vi "ShooterSpeedRegulateV2.vi"(0 "Shooter Speed":T1(ring)) -> (4 "ALL GOOD":bool, 10 "Motor 1 Output":dbl)   [LabVIEW 2012]
uses:
  Robot Global Data.vi
  Max'sToolKit/ConvertVoltageToPercentVbs.vi
  <vilib>/addons/control/pid/pid.llb/PID (DBL).vi
  <vilib>/addons/control/pid/NI_PID_pid.lvlib
panel:
  in  "Reset Shooter PID":bool
  out "Loop Rate (Hz)":dbl
  out "Array Index":dbl
  out "Wheel 1 RPS":dbl
  out "W1 Target RPS":dbl
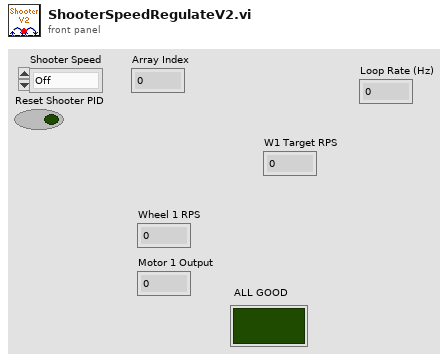
[diagram p1: front panel]
types:
  T1 = enum16{"Off", "2pt Key Shot", "3pt Key Shot", "Back Shot", "Fender Shot", "Key Close", "Key Far"}
  T2 = typedef "WPI_EncoderDevRef.ctl" = cluster{"DevStatus":errorcluster, "EncoderIndex":T3, "CounterIndex":T4, "DistancePerCount":dbl, "Decoding Type":T5}
  T3 = typedef "FPGA_EncoderIdx.ctl" = enum8{"Enc 0", "Enc 1", "Enc 2", "Enc 3", "Invalid"}
  T4 = typedef "FPGA_CounterCtrSystemIndex.ctl" = enum8{"Ctr 0", "Ctr 1", "Ctr 2", "Ctr 3", "Ctr 4", "Ctr 5", "Ctr 6", "Ctr 7", "Invalid"}
  T5 = typedef "WPI_EncoderType.ctl" = enum16{"1x", "2x", "4x"}
  T6 = cluster{"proportional gain (Kc)":dbl, "integral time (Ti, min)":dbl, "derivative time (Td, min)":dbl}
  T7 = typedef "WPI_MotorControlDeviceRef.ctl" = cluster{"DeviceStatus":errorcluster, "Type":enum16{"PWM", "CAN"}, "PWM":cluster{"Digital Module":T8, "PWM Channel":T9, "DeadBand":T10}, "CAN":cluster{"Device Number":u8, "Control Mode":T11, "Semaphore":T12, "Max Vout":dbl}, "Invert":bool, "TransformRef":T13, "InvTransformRef":T13}
  T8 = typedef "FPGA_TypedefDigitalModule.ctl" = enum16{"Digital Module 1", "Digital Module 2"}
  T9 = typedef "FPGA_DIOPWMChannel.ctl" = enum8{"PWM 1", "PWM 2", "PWM 3", "PWM 4", "PWM 5", "PWM 6", "PWM 7", "PWM 8", "PWM 9", "PWM 10", "Invalid"}
  T10 = typedef "WPI_PWMDeadband.ctl" = cluster{"Name":string, "maxPositivePwm":i32, "minPositivePwm":i32, "centerPwm":i32, "maxNegativePwm":i32, "minNegativePwm":i32, "angularRange":u16}
  T11 = typedef "WPI_CANJaguar_ControlMode.ctl" = enum8{"Percent VBus", "Current", "Speed", "Position", "Voltage"}
  T12 = typedef "Semaphore RefNum" = refnum<k1>
  T13 = typedef "WPI_PWMTransform_ConPane.ctl" = refnum<vi>
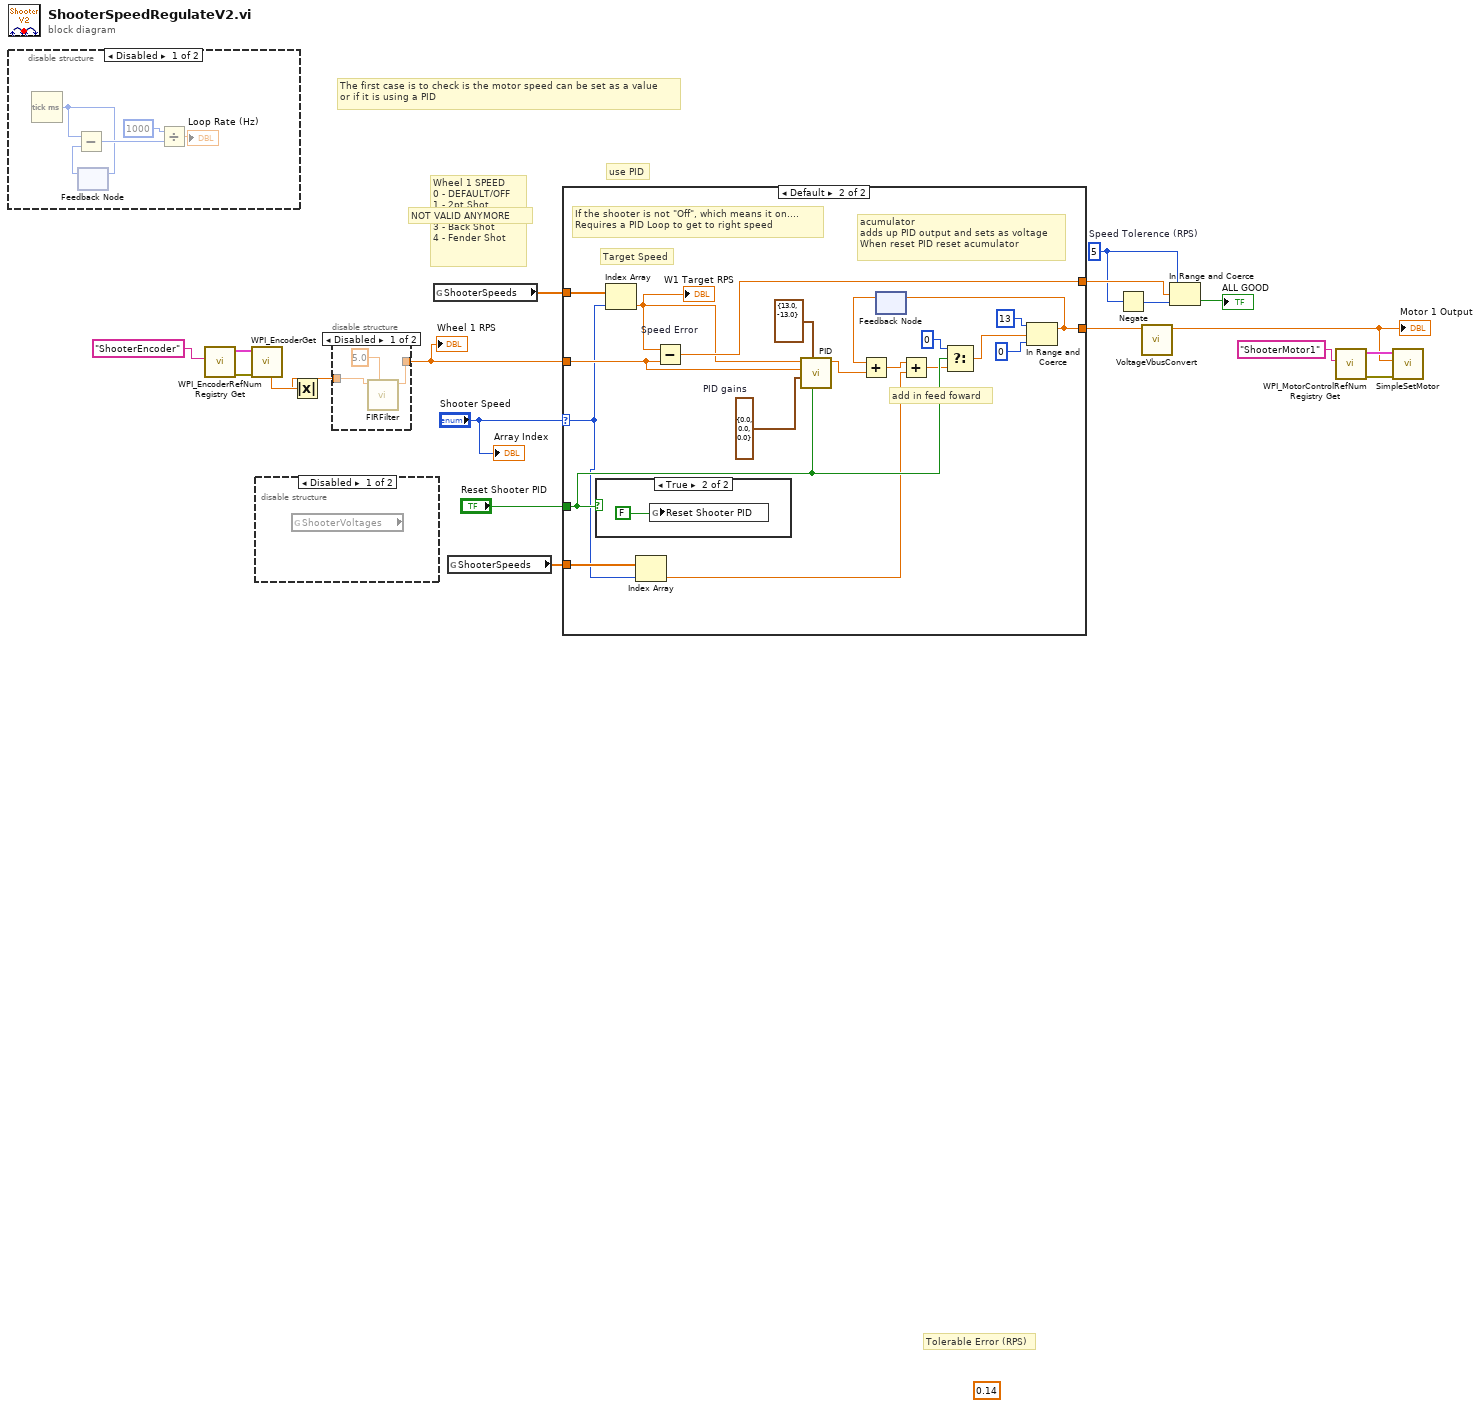
[diagram p0: block diagram]
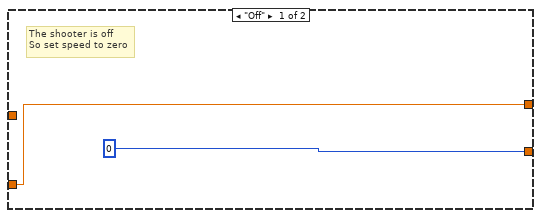
[diagram p5: hidden frame]
diagram:
  w4 = 5  # Speed Tolerence (RPS)
  (unwired) 0.14
  # "use PID"
  # "NOT VALID ANYMORE"
  # "The first case is to check is the motor speed can be set as a value\nor if it is using a PID"
  # "Tolerable Error (RPS)"
  # "Wheel 1 SPEED\n0 - DEFAULT/OFF\n1 - 2pt Shot\n2 - 3pt Key Shot\n3 - Back Shot\n4 - Fender Shot"
  n1 = disable-structure shown="Disabled" {
    frame Disabled {
      n2 = Tick Count (ms)() -> (millisecond timer value=w20:u32)
      n3 = feedback #1() -> (w21:u32)  [unwired: 1 in]
      n4 = Subtract(x=w20, y=w21) -> (x-y=w23:u32)
      n5 = feedback-in #1(w20) -> ()
      n6 = Divide(x=1000, y=w23) -> (x/y=→"Loop Rate (Hz)":dbl)
    }
    frame Enabled {
    }
  }
  n7 = call <vilib>:"WPI_EncoderRefNum Registry Get.vi"("refnum name"="ShooterEncoder") -> ("error out"=w11:errorcluster, "EncoderDevRef"=w12:T2)  [unwired: 9 in]
  n8 = call <vilib>:"WPI_EncoderGet.vi"("error in (no error)"=w11, "EncoderDevRef"=w12) -> ("Rate"=w8:dbl)  [unwired: 4 in, 5 out]
  n9 = disable-structure shown="Disabled" {
    frame Disabled {
      n10 = global read "Robot Global Data.vi" "ShooterVoltages"() -> ()  [unwired: 1 out]
    }
    frame Enabled {
    }
  }
  n11 = Absolute Value(x=w8) -> (abs(x)=w7:dbl)
  n12 = disable-structure shown="Disabled" {
    disable-tunnel: [w26 w28] -> w10
    disable-tunnel: w7 -> [w25 w28]
    frame Disabled {
      n13 = call "FIRFilter.vi"("Filter Size"=5.0 ("Filter size"), "Input"=w25) -> ("Output"=w26:dbl)  [unwired: 9 in]
    }
    frame Enabled {
    }
  }
  "Wheel 1 RPS" <- w10
  n14 = global read "Robot Global Data.vi" "ShooterSpeeds"() -> (w9:dbl[])
  n15 = global read "Robot Global Data.vi" "ShooterSpeeds"() -> (w1:dbl[])
  n16 = case shown="Default" "Shooter Speed" {
    selector: "Shooter Speed" -> [_ w35]
    tunnel: w10 -> [w29 w43]
    tunnel: [0 w46] -> w3
    tunnel: [w29 w44] -> w14
    tunnel: w9 -> [_ w41]
    tunnel: "Reset Shooter PID" -> [_ w38]
    tunnel: w1 -> [_ w36]
    frame "Off" {
      # "The shooter is off\nSo set speed to zero"
    }
    frame Default {
      w45 = T6 {"proportional gain (Kc)"=0.0, "integral time (Ti, min)"=0.0, "derivative time (Td, min)"=0.0}  # PID gains
      # "add in feed foward"
      # "acumulator\nadds up PID output and sets as voltage\nWhen reset PID reset acumulator"
      # "Target Speed"
      # "If the shooter is not \"Off\", which means it on....\nRequires a PID Loop to get to right speed"
      n17 = case shown="True" w38 {
        frame False {
        }
        frame True {
          n18 = global write "Robot Global Data.vi" "Reset Shooter PID"(FALSE) -> ()
        }
      }
      n19 = Index Array(array=w41, index=w35) -> (element=w39:dbl)
      "W1 Target RPS" <- w39
      n20 = Index Array(array=w36, index=w35) -> (element=w33:dbl)
      n21 = Subtract "Speed Error"(x=w39, y=w43) -> (x-y=w44:dbl)
      n22 = call-poly <vilib>:"PID.vi"("reinitialize? (F)"=w38, "output range"=cluster{"output high":dbl, "output low":dbl} {"output high"=13.0, "output low"=-13.0}, "PID gains"=w45, "process variable"=w43, "setpoint"=w39) -> ("output"=w37:dbl)  [unwired: 5 in, 1 out]
      n23 = feedback #2() -> (w40:dbl)  [unwired: 1 in]
      n24 = Add(x=w40, y=w37) -> (x+y=w32:dbl)
      n25 = Add(x=w32, y=w33) -> (x+y=w31:dbl)
      n26 = Select(t=0, s=w38, f=w31) -> (s? t:f=w34:dbl)
      n27 = In Range and Coerce(upper limit=13, x=w34, lower limit=0 ("upper limit")) -> (coerced(x)=w46:dbl)  [unwired: 1 out]
      n28 = feedback-in #2(w46) -> ()
    }
  }
  n29 = Negate(x=w4) -> (-x=w15:i32)
  n30 = call-poly "VoltageVbusConvert.vi"("Voltage"=w3) -> ("Vbus"=w2:dbl)  [unwired: 10 in]
  "Motor 1 Output" <- w2
  n31 = In Range and Coerce(upper limit=w4, x=w14, lower limit=w15) -> (In Range?=→"ALL GOOD":bool)  [unwired: 1 out]
  n32 = call <vilib>:"WPI_MotorControlRefNum Registry Get.vi"("refnum name"="ShooterMotor1") -> ("error out"=w17:errorcluster, "MotorControlDevRef"=w18:T7)  [unwired: 9 in]
  n33 = call "SimpleSetMotor.vi"("error in (no error)"=w17, "Output"=w2, "MotorControlDevRef"=w18) -> ()  [unwired: 7 in, 2 out]
  "Array Index" <- "Shooter Speed"
